vi "Hypot.vi"() -> ()   [LabVIEW 2018]
panel:
  out "Output":dbl
  in  "Y":dbl
  in  "X":dbl
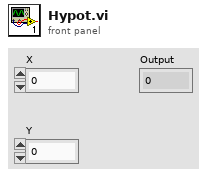
[diagram p1: front panel]
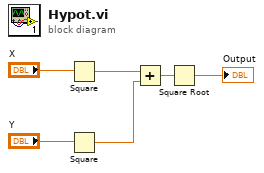
[diagram p0: block diagram]
diagram:
  n1 = Square(x="X") -> (x^2=w6:dbl)
  n2 = Square(x="Y") -> (x^2=w5:dbl)
  n3 = Add(x=w6, y=w5) -> (x+y=w4:dbl)
  n4 = Square Root(x=w4) -> (sqrt(x)=→"Output":dbl)
